vi "Temp_Generator.vi"(0 "Highest_Sys_Temp":dbl=100.0, 5 "Lowest_Sys_Temp":dbl) -> (4 "Temp":dbl)   [LabVIEW 2023]
uses:
  <vilib>/numeric/Random Number (Range) DBL.vi
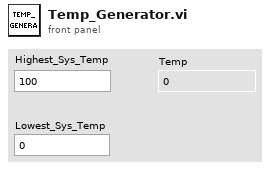
[diagram p1: front panel]
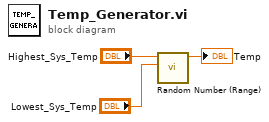
[diagram p0: block diagram]
diagram:
  n1 = call-poly <vilib>:"Random Number (Range).vi"("lower bound (0)"="Lowest_Sys_Temp", "upper bound (100)"="Highest_Sys_Temp") -> ("number"=→"Temp":dbl)  [unwired: 9 in]
